vi "AVItoColorImageToArray.vi"() -> ()   [LabVIEW 2017]
uses:
  <vilib>/Utility/file.llb/Write To Spreadsheet File (I64).vi
panel:
  in  "AVI Path":path=path "C:/Documents and Settings/ravikant/Desktop/ArrayToAVI/5.avi"
  in  "String":string="AVIimage5_"
  out "Image":T1(plugin-control)
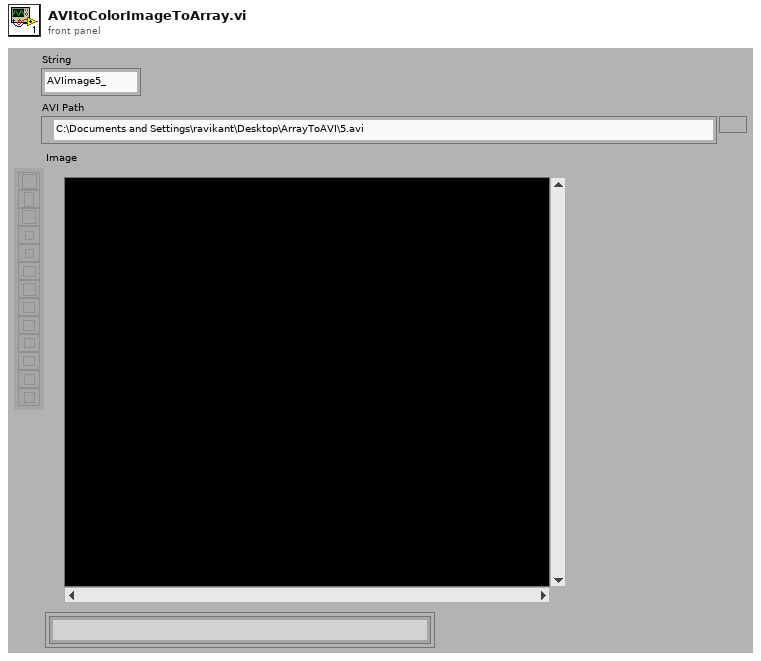
[diagram p1: front panel]
types:
  T1 = typedef "IMAQ Image.ctl" = refnum<image>
  T2 = typedef "Image Type" = u32
  T3 = typedef "AviRefnum.ctl" = refnum<k1>
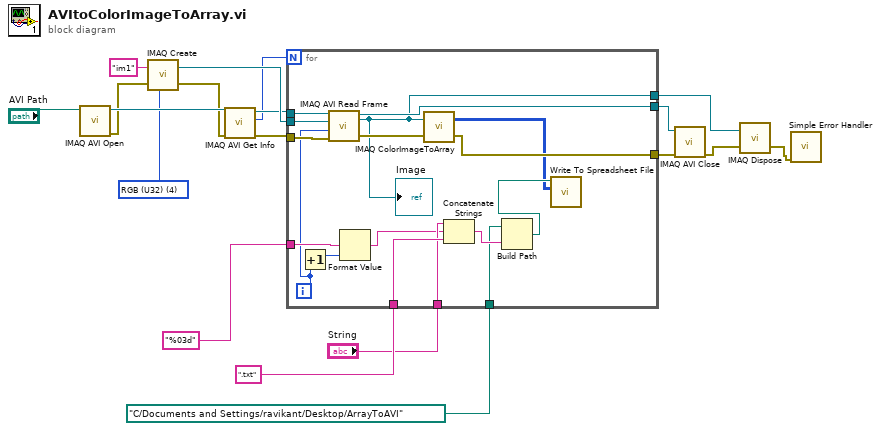
[diagram p0: block diagram]
diagram:
  w5 = T2 4 items=["Grayscale (U8)", "Grayscale (I16)", "Grayscale (SGL)", "Complex (CSG)", "RGB (U32)", "HSL (U32)", "RGB (U64)"] ("Image Type")
  n1 = call "IMAQ AVI Open"("AVI Path"="AVI Path") -> ("error out"=w1:errorcluster, "Avi Refnum"=w16:T3)  [unwired: 9 in]
  n2 = call "IMAQ Create"("Image Name"="im1", "Image Type"=w5, "error in (no error)"=w1) -> ("New Image"=w18:T1, "error out"=w15:errorcluster)  [unwired: 2 in]
  n3 = call "IMAQ AVI Get Info"("error in (no error)"=w15, "Avi Refnum"=w16) -> ("error out"=w14:errorcluster, "Number of Frames"=w8:u32, "Avi Refnum (duplicate)"=w13:T3)  [unwired: 5 in, 2 out]
  n4 = for {
    N: w8 -> [_]
    tunnel: w18 -> [w36]
    tunnel: w14 -> [w35]
    tunnel: w13 -> [w34]
    tunnel: path "C:/Documents and Settings/ravikant/Desktop/ArrayToAVI" ("base path") -> [w30]
    tunnel: ".txt" -> [w29]
    tunnel: "%03d" -> [w27]
    tunnel: "String" -> [w26]
    tunnel: [w23] -> w7
    tunnel: [w22] -> w6
    tunnel: [w21] -> w4
    i -> [w24]
    n5 = Increment(x=w24) -> (x+1=w28:i32)
    n6 = call "IMAQ AVI Read Frame"("error in (no error)"=w35, "Frame Number"=w24, "Image"=w36, "Avi Refnum"=w34) -> ("error out"=w33:errorcluster, "Image Out"=w21:T1, "Avi Refnum (duplicate)"=w22:T3)  [unwired: 4 in, 1 out]
    "Image" <- w21
    n7 = Format Value(format string=w27, value (0)=w28) -> (output string=w25:string)  [unwired: 1 in]
    n8 = call "IMAQ ColorImageToArray"("Image"=w21, "error in (no error)"=w33) -> ("Image Pixels (U32)"=w20:u32[][], "error out"=w23:errorcluster)  [unwired: 2 in, 1 out]
    n9 = Concatenate Strings(w26, w25, w29) -> (w32:string)
    n10 = Build Path(base path=w30, name or relative path=w32) -> (appended path=w31:path)
    n11 = call-poly <vilib>:"Write To Spreadsheet File.vi"("2D data"=w20, "file path (dialog if empty)"=w31) -> ()  [unwired: 6 in, 1 out]
  }
  n12 = call "IMAQ AVI Close"("error in (no error)"=w7, "Avi Refnum"=w6) -> ("error out"=w3:errorcluster)  [unwired: 9 in]
  n13 = call "IMAQ Dispose"("Image"=w4, "error in (no error)"=w3) -> ("error out"=w2:errorcluster)  [unwired: 4 in]
  n14 = call <vilib>:"Simple Error Handler.vi"("error in (no error)"=w2) -> ()  [unwired: 4 in, 5 out]
